vi "getStateValue.vi"(8 "error in (no error)":errorcluster, 11 "rf in":refnum<class "rf.lvclass">) -> (0 "error out":errorcluster, 2 "stateValue":string, 3 "rf out":refnum<class "rf.lvclass">)   [LabVIEW 2009, in "Tools.lvlib" / "Scripting.lvlib" / "rf.lvclass"]
uses:
  rf.lvclass
  ScriptEvent.lvclass
  DatabaseHelpers/Database Objects/Channel/RfOutputChannel/RfOutputChannel.lvclass
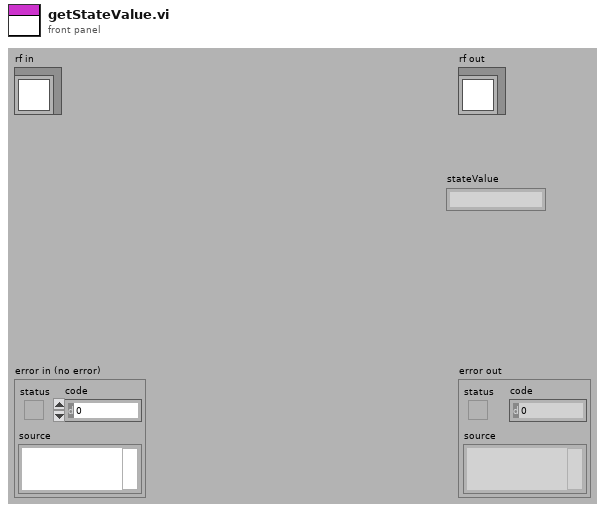
[diagram p1: front panel]
types:
  T1 = cluster{"state_name":string, "value":cluster{"frequency":string, "amplitude":string, "phase":string}}[]
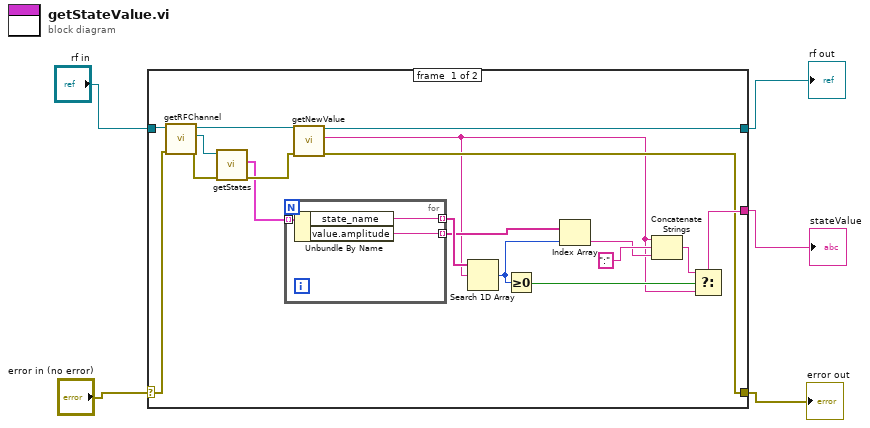
[diagram p0: block diagram]
diagram:
  n1 = case shown="No Error" "error in (no error)" {
    selector: "error in (no error)" -> [w18 w28]
    tunnel: [w10 w28] -> w3
    tunnel: [w9 w27] -> w1
    tunnel: "rf in" -> [w19 w27]
    tunnel: [w20 _] -> w2
    frame #0 {
      n2 = call "getRFChannel.vi"("error in (no error)"=w18, "rf.lvclass in"=w19) -> ("error out"=w16:errorcluster, "RfOutputChannel.lvclass"=w17:refnum<class "RfOutputChannel.lvclass">, "rf.lvclass out"=w15:refnum<class "rf.lvclass">)  [unwired: 7 in]
      n3 = call "getStates.vi"("error in (no error)"=w16, "RfOutputChannel in"=w17) -> ("error out"=w14:errorcluster, "states"=w13:T1)  [unwired: 7 in, 1 out]
      n4 = for {
        tunnel: w13 -> [w26] mode=indexing
        tunnel: [w25] -> w12 mode=indexing
        tunnel: [w24] -> w8 mode=indexing
        n5 = Unbundle By Name(w26) -> ("state_name"=w25:string, "value.amplitude"=w24:string)
      }
      n6 = call "getNewValue.vi"("error in (no error)"=w14, "ScriptEvent.lvclass in"=w15) -> ("error out"=w10:errorcluster, "newValue"=w6:string, "ScriptEvent.lvclass out"=w9:refnum<class "rf.lvclass">)  [unwired: 7 in]
      n7 = Search 1D Array(1D array=w12, element=w6) -> (index of element=w11:i32)  [unwired: 1 in]
      n8 = Greater Or Equal To 0?(x=w11) -> (x >= 0?=w21:bool)
      n9 = Index Array(array=w8, index=w11) -> (element=w7:string)
      n10 = Concatenate Strings(w6, ":", w7) -> (w22:string)
      n11 = Select(t=w22, s=w21, f=w6) -> (s? t:f=w20:string)
    }
    frame #1 {
    }
  }
  "error out" <- w3
  "rf out" <- w1
  "stateValue" <- w2
